vi "ukol2.vi"() -> ()   [LabVIEW 2023]
uses:
  <vilib>/Analysis/2dsp.llb/1D Convolution (DBL).vi
  <vilib>/Utility/file.llb/Read Delimited Spreadsheet (DBL).vi
  <vilib>/Analysis/NI_AALBase.lvlib
  <vilib>/Analysis/NI_AALPro.lvlib
panel:
  out "Waveform Graph 3":dbl[](graph)
  out "Waveform Graph 2":dbl[](graph)
  out "Waveform Graph":dbl[](graph)
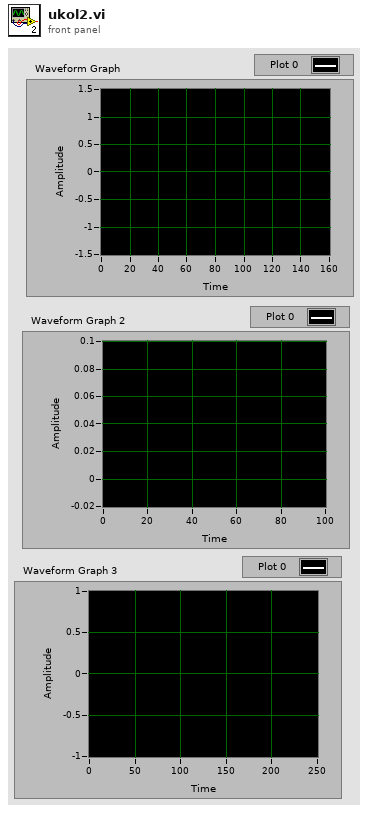
[diagram p1: front panel]
types:
  T1 = cluster{"frequency":dbl, "amplitude":dbl, "phase":dbl}[]
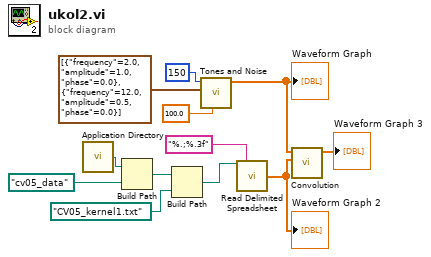
[diagram p0: block diagram]
diagram:
  n1 = call <vilib>:"Application Directory.vi"() -> ("Application Directory"=w9:path)
  n2 = Build Path(base path=w9, name or relative path=path "cv05_data") -> (appended path=w7:path)
  n3 = Build Path(base path=w7, name or relative path=path "CV05_kernel1.txt") -> (appended path=w5:path)
  n4 = call <vilib>:"Tones and Noise.vi"("Fs"=100.0, "tones"=T1 [{"frequency"=2.0, "amplitude"=1.0, "phase"=0.0}, {"frequency"=12.0, "amplitude"=0.5, "phase"=0.0}], "samples"=150) -> ("tones and noise"=w3:dbl[])  [unwired: 7 in, 1 out]
  "Waveform Graph" <- w3
  n5 = call-poly <vilib>:"Read Delimited Spreadsheet.vi"("file path (dialog if empty)"=w5, "format (%.3f)"="%.;%.3f") -> ("first row"=w1:dbl[])  [unwired: 8 in, 5 out]
  "Waveform Graph 2" <- w1
  n6 = call-poly <vilib>:"Convolution.vi"("Y"=w1, "X"=w3) -> ("X * Y"=→"Waveform Graph 3":dbl[])  [unwired: 8 in, 1 out]
